vi "PCA CreateEmpty.vi"(8 "error in (no error)":errorcluster) -> (0 "error out":errorcluster, 3 "PCA out":refnum<class "PCA.lvclass">)   [LabVIEW 2020, in "OpenLvVision_OpenCv.lvlib" / "PCA.lvclass"]
doc: "Object by reference!\nThe default constructor initializes an empty PCA structure. The other constructors initialize the structure ."
uses:
  PCA.lvclass
  C:/Users/lukas/Downloads/OpenLvVision_OpenCv/SourceCode/LabView/OpenLvVision_OpenCv/_LvHelpers/EdvrObject/EdvrObject.lvclass
  _LvHelpers/EdvrObject/TypeDef/Edvr.ctl
  _LvHelpers/EdvrObject/EdvrObject.lvclass/EdvrObject.ctl
  _LvHelpers/EdvrObject/EdvrObject.lvclass
  OpenLvVision_OpenCv.lvlib
  Dlls/OlvOpenCvWrapper.dll
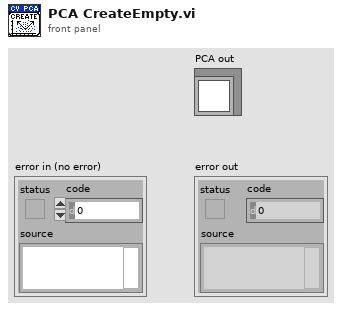
[diagram p1: front panel]
types:
  T1 = typedef "OpenLvVision_OpenCv.lvlib/EdvrObject.lvclass/Edvr.ctl" = refnum<data-value>
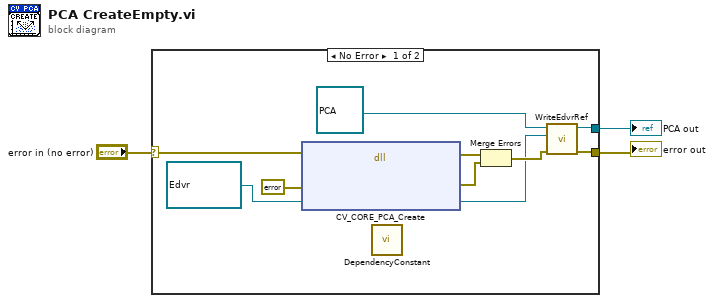
[diagram p0: block diagram]
diagram:
  n1 = case shown="No Error" "error in (no error)" {
    selector: "error in (no error)" -> [w10 w14]
    tunnel: [w12 w14] -> w1
    tunnel: [w13 _] -> w2
    frame No Error {
      n2 = dll-call lib="C:/Users/lukas/Downloads/OpenLvVision_OpenCv/SourceCode/LabView/OpenLvVision_OpenCv/Dlls/OlvOpenCvWrapper.dll" fn="CV_CORE_PCA_Create"(error in=w10, "Error"=errorcluster {"status"=FALSE, "code"=0, "source"=""} ("error out"), "edvrRef"=T1 refnum ("Edvr")) -> (error out=w8:errorcluster, "Error"=w5:errorcluster, "edvrRef"=w6:T1)  [unwired: 3 in, 1 out]
      n3 = call "DependencyConstant.vi"() -> ()  [unwired: 12 in]
      n4 = Merge Errors(w8, w5) -> (w7:errorcluster)
      n5 = call "WriteEdvrRef.vi"("error in (no error)"=w7, "Edvr"=w6, "EdvrObject in"=refnum<class "PCA.lvclass"> refnum ("OpenLvVision_OpenCv.lvlib:PCA")) -> ("error out"=w12:errorcluster, "EdvrObject out"=w13:refnum<class "PCA.lvclass">)  [unwired: 7 in]
    }
    frame Error {
    }
  }
  "error out" <- w1
  "PCA out" <- w2
